vi "Create Channel Headers.vi"(8 "错误输入":cluster{"状态":bool, "代码":i32, "源":string}, 9 "通道名":string[](array[string]), 11 "文件引用句柄输入":refnum<file>) -> (0 "错误输出":cluster{"状态":bool, "代码":i32, "源":string}, 3 "文件引用句柄输出":refnum<file>)   [LabVIEW 2012]
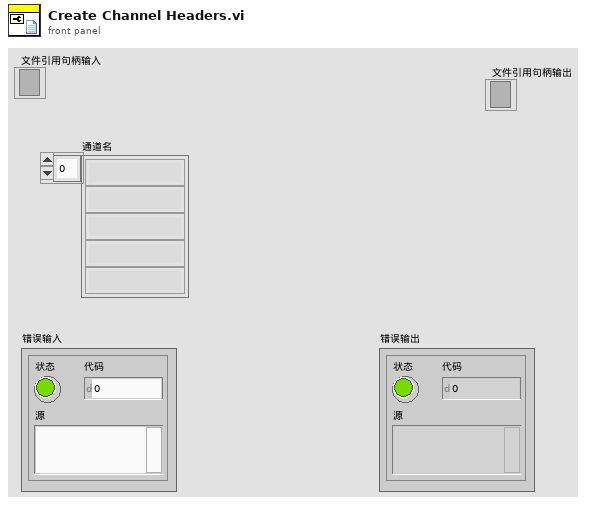
[diagram p1: front panel]
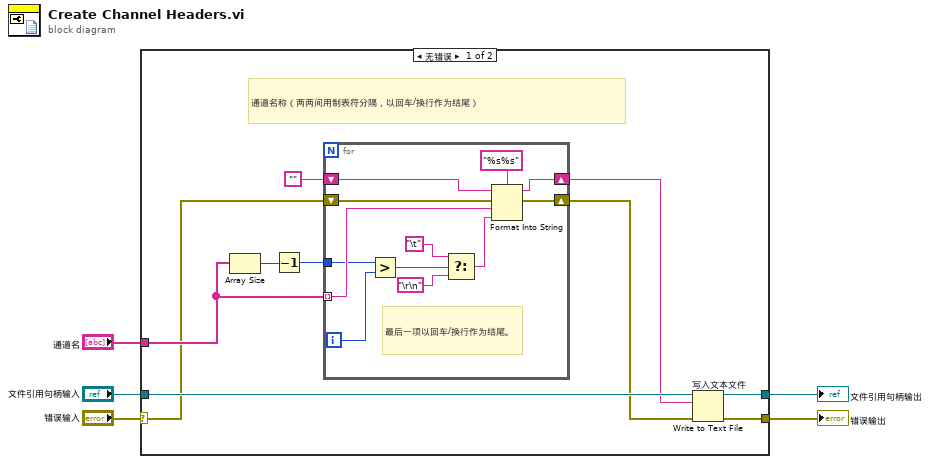
[diagram p0: block diagram]
diagram:
  n1 = case shown="无错误" "错误输入" {
    selector: "错误输入" -> [w7 w28]
    tunnel: [w13 w28] -> w3
    tunnel: "文件引用句柄输入" -> [w15 w29]
    tunnel: [w14 w29] -> w4
    tunnel: "通道名" -> [w10 _]
    frame No Error {
      # "通道名称（两两间用制表符分隔，以回车/换行作为结尾）"
      n2 = Array Size ("数组大小")(array=w10) -> (size(s)=w12:i32)
      n3 = Decrement ("减1")(x=w12) -> (x-1=w11:i32)
      n4 = for {
        shift-right: [w26] -> w8
        shift-left: "" ("空字符串常量") -> [w27]
        tunnel: w10 -> [w25] mode=indexing
        shift-right: [w23] -> w6
        shift-left: w7 -> [w24]
        tunnel: w11 -> [w18]
        i -> [w17]
        # "最后一项以回车/换行作为结尾。"
        n5 = Greater? ("大于？")(x=w18, y=w17) -> (0:w16:bool)
        n6 = Select ("选择")(t="\t" ("制表符常量"), s=w16, f="\r\n" ("行结束常量")) -> (s? t:f=w21:string)
        n7 = Format Into String ("格式化写入字符串")(format string="%s%s" ("格式字符串"), initial string=w27, error in=w24, w25, w21) -> (resulting string=w26:string, error out=w23:errorcluster)
      }
      n8 = Write to Text File "写入文本文件"(file (use dialog)=w15, text=w8, error in=w6) -> (refnum out=w14:refnum<file>, error out=w13:errorcluster)  [unwired: 1 in, 1 out]
    }
    frame Error {
    }
  }
  "文件引用句柄输出" <- w4
  "错误输出" <- w3
